vi "vi.ChangeSettings.vi"() -> ()   [LabVIEW 2014]
panel:
  out "Numeric":i32
  out "array w/ subset deleted":string[](array[string])
  out "appended path":path
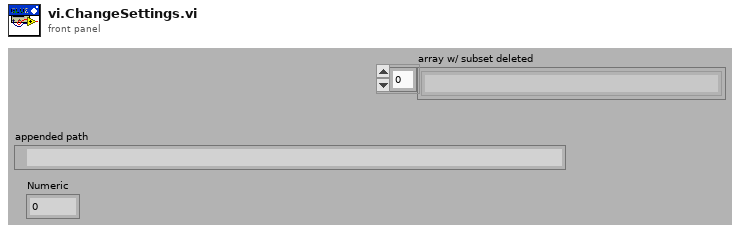
[diagram p1: front panel]
types:
  T1 = enum32{"invalid priority", "background priority", "normal priority", "above normal priority", "high priority", "time critical priority", "subroutine"}
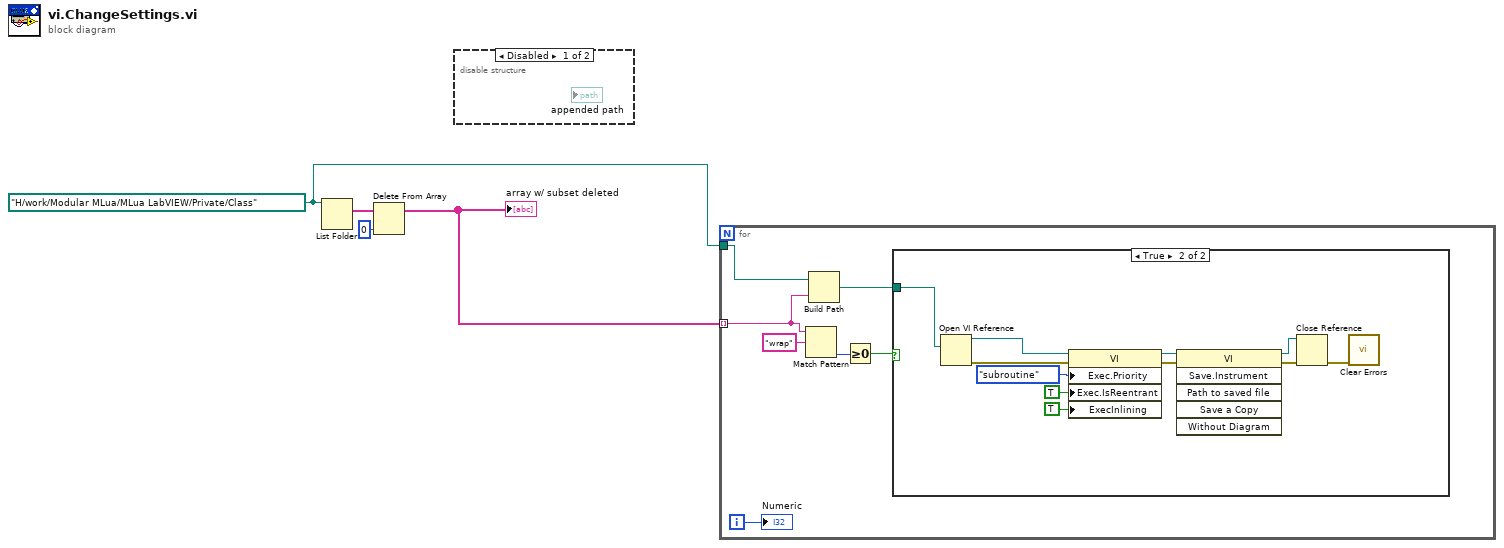
[diagram p0: block diagram]
diagram:
  w1 = path "H:/work/Modular MLua/MLua LabVIEW/Private/Class" ("path")
  n1 = List Folder(path=w1) -> (filenames=w4:string[])  [unwired: 3 in, 3 out]
  n2 = Delete From Array(array=w4, index=0) -> (array with subset deleted=w2:string[])  [unwired: 1 in, 1 out]
  "array w/ subset deleted" <- w2
  n3 = disable-structure shown="Disabled" {
    frame Disabled {
    }
    frame Enabled {
    }
  }
  n4 = for {
    tunnel: w2 -> [w8] mode=indexing
    tunnel: w1 -> [w9]
    i -> [w5]
    n5 = Match Pattern(string=w8, regular expression="wrap") -> (offset past match=w11:i32)  [unwired: 1 in, 3 out]
    n6 = Build Path(base path=w9, name or relative path=w8) -> (appended path=w6:path)
    n7 = Greater Or Equal To 0?(x=w11) -> (x >= 0?=w7:bool)
    n8 = case shown="True" w7 {
      tunnel: w6 -> [_ w12]
      frame False {
      }
      frame True {
        n9 = Open VI Reference(vi path=w12) -> (vi reference=w22:refnum<vi>, error out=w21:errorcluster)  [unwired: 5 in]
        n10 = property class="VI"(reference=w22, error in=w21, "Exec.Priority"=T1."subroutine" ("Execution:Priority"), "Exec.IsReentrant"=TRUE ("Execution:Is Reentrant"), "ExecInlining"=TRUE ("Execution:Inline SubVI")) -> (reference out=w16:refnum<vi>, error out=w17:errorcluster)
        n11 = invoke class="VI" method="Save.Instrument"(reference=w16, error in=w17) -> (reference out=w14:refnum<vi>, error out=w15:errorcluster)  [unwired: 4 in, 4 out]
        n12 = Close Reference(reference=w14, error in (no error)=w15) -> (error out=w13:errorcluster)
        n13 = call <vilib>:"Clear Errors.vi"("error in (no error)"=w13) -> ()  [unwired: 5 in, 2 out]
      }
    }
    "Numeric" <- w5
  }
